vi "AdvanceTable_InitData.vi"(6 "NumInPage":u32, 7 "NumOfUnsaw":u32, 8 "error in (no error)":errorcluster, 9 "Scroller.lvclass":refnum<class "Scroller.lvclass">, 10 "Items":refnum<class "TableItem.lvclass">[](array[class]), 11 "object in":refnum<class "AdvanceTable.lvclass">) -> (0 "error out":errorcluster, 3 "object out":refnum<class "AdvanceTable.lvclass">)   [LabVIEW 2015, in "ActorManagement.lvlib" / "AdvanceTable.lvclass"]
uses:
  AdvanceTable.lvclass
  TableItem/TableItem.lvclass
  Scroll/Scroller.lvclass
  AdvanceTable.lvclass/AdvanceTable.ctl
  Config/g_tabSetting.vi
  ActorManagement.lvlib
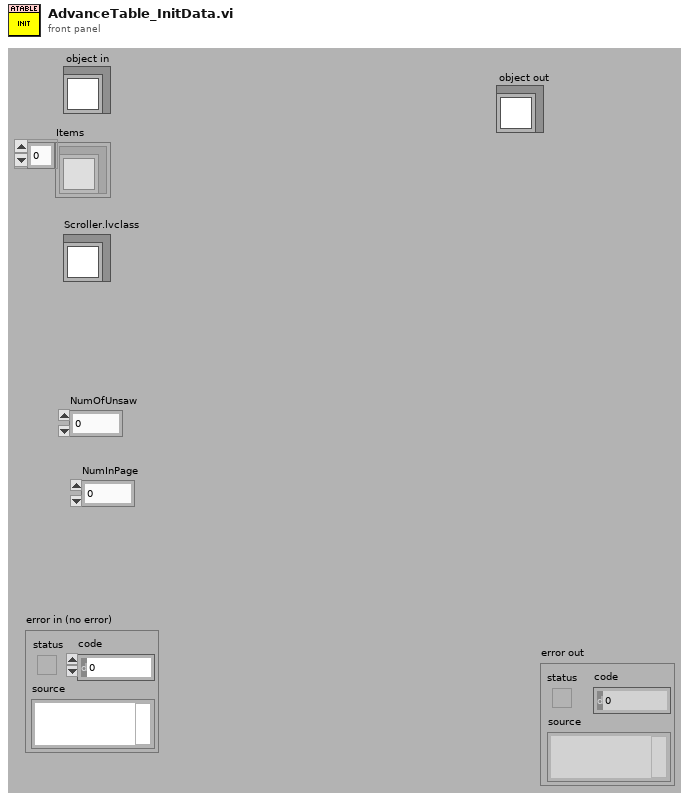
[diagram p1: front panel]
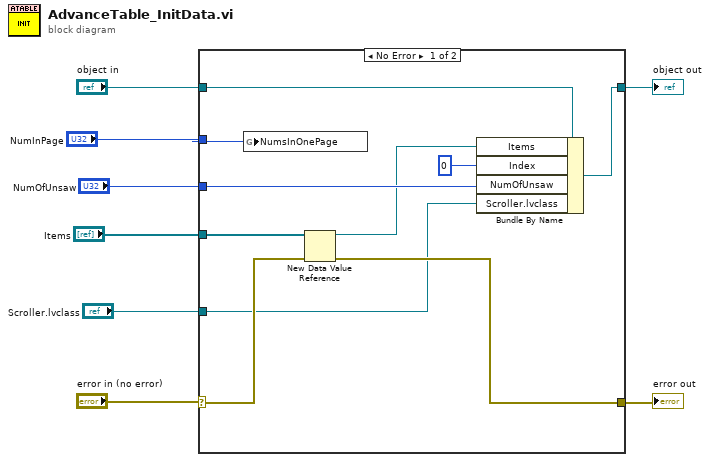
[diagram p0: block diagram]
diagram:
  n1 = case shown="No Error" "error in (no error)" {
    selector: "error in (no error)" -> [w13 w19]
    tunnel: "object in" -> [w18 w20]
    tunnel: [w17 w20] -> w7
    tunnel: [w12 w19] -> w5
    tunnel: "Items" -> [w15 _]
    tunnel: "NumInPage" -> [w9 _]
    tunnel: "NumOfUnsaw" -> [w16 _]
    tunnel: "Scroller.lvclass" -> [w11 _]
    frame No Error {
      n2 = global write "g_tabSetting.vi" "NumsInOnePage"(w9) -> ()
      n3 = New Data Value Reference(data value=w15, error in=w13) -> (data value reference=w14:refnum<data-value>, error out=w12:errorcluster)
      n4 = Bundle By Name(cluster=w18, "Items"=w14, "Index"=u32 0, "NumOfUnsaw"=w16, "Scroller.lvclass"=w11) -> (w17:refnum<class "AdvanceTable.lvclass">)
    }
    frame Error {
    }
  }
  "object out" <- w7
  "error out" <- w5
